vi "Close.vi"(8 "error in (no error)":errorcluster, 11 "KE27XX DMM in":refnum<class "Keithley 27XX DMM.lvclass">) -> (0 "error out":errorcluster, 3 "KE27XX DMM out":refnum<class "Keithley 27XX DMM.lvclass">)   [LabVIEW 2025, in "DMM.lvlib" / "Keithley 27XX DMM.lvclass"]
uses:
  Keithley 27XX DMM.lvclass
  Keithley 27XX DMM.lvclass/Keithley 27XX DMM.ctl
  <instrlib>/Keithley 27XX/Keithley 27XX.lvlib
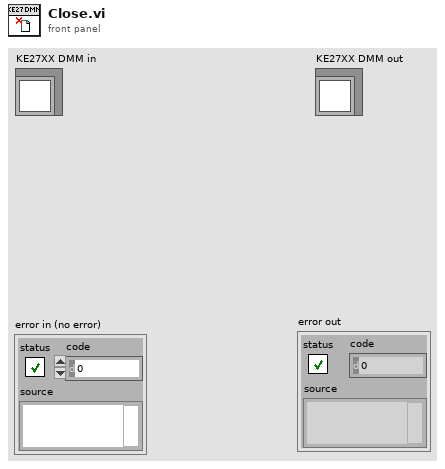
[diagram p1: front panel]
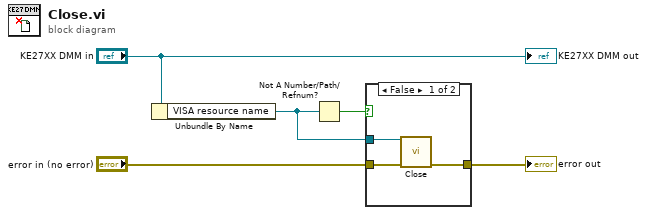
[diagram p0: block diagram]
diagram:
  n1 = Unbundle By Name("KE27XX DMM in") -> ("VISA resource name"=w3:refnum<visa-resource-name>)
  n2 = Not A Number/Path/Refnum?(number/path/refnum=w3) -> (NaN/Path/Refnum?=w2:bool)
  n3 = case shown="False" w2 {
    tunnel: "error in (no error)" -> [w8 w9]
    tunnel: [w7 w9] -> w4
    tunnel: w3 -> [w6 _]
    frame False {
      n4 = call <instrlib>:"Close.vi"("VISA resource name"=w6, "error in (no error)"=w8) -> ("error out"=w7:errorcluster)  [unwired: 13 in]
    }
    frame True {
    }
  }
  "error out" <- w4
  "KE27XX DMM out" <- "KE27XX DMM in"
